vi "Is Empty.vi"(8 "error in (no error)":errorcluster, 11 "Tag_LVOOP in":refnum<class "Tree Tag Class.lvclass">) -> (0 "error out":errorcluster, 2 "Empty":bool, 3 "Tag_LVOOP out":refnum<class "Tree Tag Class.lvclass">)   [LabVIEW 2012, in "Tree Tools.lvlib" / "Tree Tag Class.lvclass"]
uses:
  Tree Tag Class.lvclass
  Tree Tag Class.lvclass/Tree Tag Class.ctl
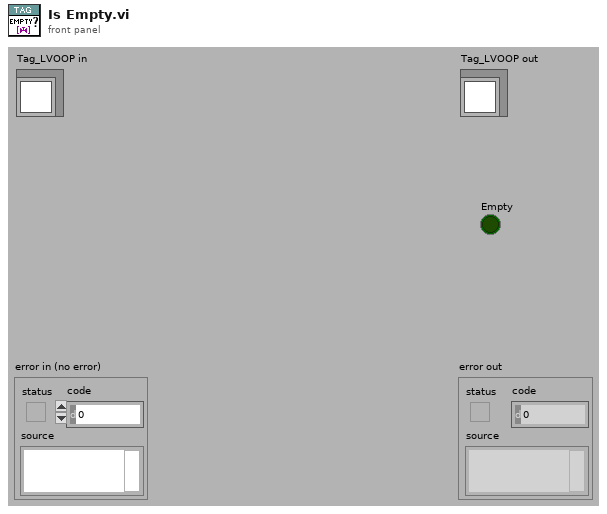
[diagram p1: front panel]
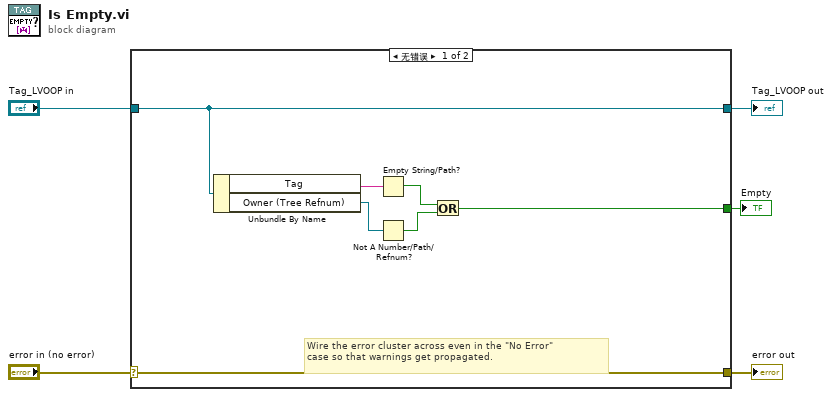
[diagram p0: block diagram]
diagram:
  n1 = case shown="无错误" "error in (no error)" {
    selector: "error in (no error)" -> [w12 w14]
    tunnel: [w12 w14] -> w4
    tunnel: [w11 w13] -> w2
    tunnel: "Tag_LVOOP in" -> [w11 w13]
    tunnel: [w6 _] -> w1
    frame No Error {
      # "Wire the error cluster across even in the \"No Error\"\ncase so that warnings get propagated."
      n2 = Unbundle By Name(w11) -> ("Tag"=w10:string, "Owner (Tree Refnum)"=w9:refnum<vi>)
      n3 = Empty String/Path?(string/path=w10) -> (empty?=w8:bool)
      n4 = Not A Number/Path/Refnum?(number/path/refnum=w9) -> (NaN/Path/Refnum?=w7:bool)
      n5 = Or(x=w8, y=w7) -> (x .or. y?=w6:bool)
    }
    frame Error {
    }
  }
  "error out" <- w4
  "Tag_LVOOP out" <- w2
  "Empty" <- w1
